vi "Random Competition.vi"() -> ()   [LabVIEW 2025]
panel:
  out "Winner B":bool
  out "Tie":bool
  out "Winner A":bool
  out "Points B":dbl
  out "Random Number B":dbl
  out "Points A":dbl
  out "Random Number A":dbl
  in  "Number of Iterations":i32
  # "ME 235: Design of Microprocessor Based Mechanical Systems"
  # "Lab 1 - Random Competition"
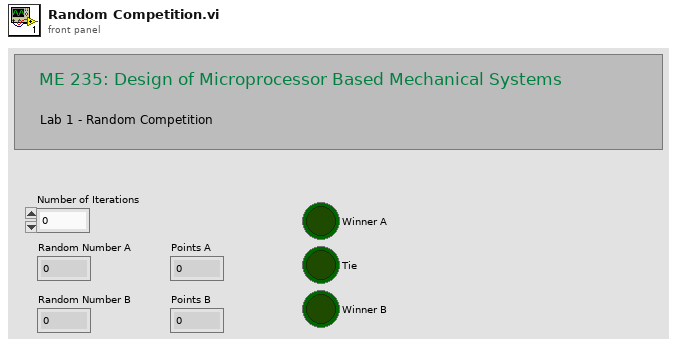
[diagram p1: front panel]
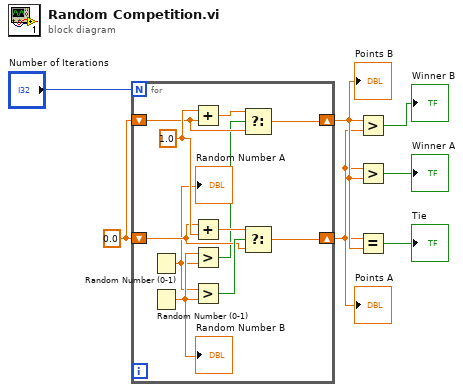
[diagram p0: block diagram]
diagram:
  w6 = 0.0
  n1 = for {
    N: "Number of Iterations" -> [_]
    shift-right: [w9] -> w2
    shift-left: w6 -> [w15]
    shift-right: [w8] -> w3
    shift-left: w6 -> [w13]
    w18 = 1.0
    n2 = Random Number (0-1)() -> (number: 0 to 1=w11:dbl)
    "Random Number A" <- w11
    n3 = Random Number (0-1)() -> (number: 0 to 1=w12:dbl)
    "Random Number B" <- w12
    n4 = Add(x=w18, y=w13) -> (x+y=w14:dbl)
    n5 = Add(x=w15, y=w18) -> (x+y=w16:dbl)
    n6 = Greater?(x=w12, y=w11) -> (0:w10:bool)
    n7 = Greater?(x=w11, y=w12) -> (0:w17:bool)
    n8 = Select(t=w14, s=w10, f=w13) -> (s? t:f=w8:dbl)
    n9 = Select(t=w16, s=w17, f=w15) -> (s? t:f=w9:dbl)
  }
  "Points A" <- w2
  "Points B" <- w3
  n10 = Greater?(x=w3, y=w2) -> (0:→"Winner B":bool)
  n11 = Greater?(x=w2, y=w3) -> (0:→"Winner A":bool)
  n12 = Equal?(x=w2, y=w3) -> (x = y?=→"Tie":bool)
